vi "18-FindLeftRightExplode.vi"(10 "Explode Position":i32, 11 "Snailfish Number in in":string) -> (0 "Right Explosion":u64, 1 "Right Snailfish Number out":string, 2 "Left Explosion":u64, 3 "Left Snailfish Number out":string)   [LabVIEW 2019, in "18.lvlib"]
uses:
  18.lvlib
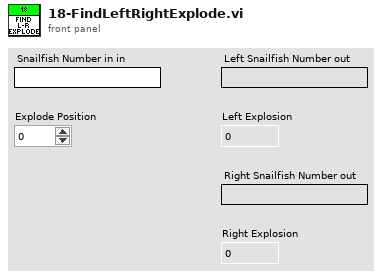
[diagram p1: front panel]
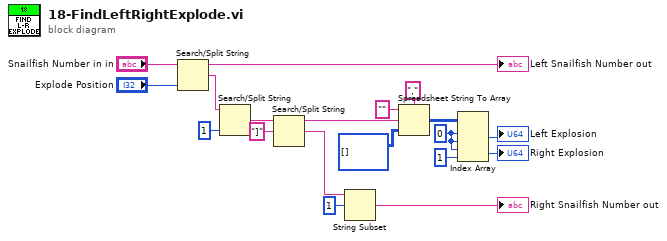
[diagram p0: block diagram]
diagram:
  w11 = 0 ("index (row)")
  n1 = Search/Split String(string="Snailfish Number in in", offset (0)="Explode Position") -> (substring before match=→"Left Snailfish Number out":string, match + rest of string=w14:string)  [unwired: 1 in, 1 out]
  n2 = Search/Split String(string=w14, offset (0)=1) -> (match + rest of string=w15:string)  [unwired: 1 in, 2 out]
  n3 = Search/Split String(string=w15, search string/char (-)="]") -> (substring before match=w6:string, match + rest of string=w3:string)  [unwired: 1 in, 1 out]
  n4 = String Subset(string=w3, offset (0)=1) -> (substring=→"Right Snailfish Number out":string)  [unwired: 1 in]
  n5 = Spreadsheet String To Array(delimiter (Tab)=",", format string="", spreadsheet string=w6, array type (2D Dbl)=u64[][] [] ("Position of Last Number")) -> (array=w10:u64[][])
  n6 = Index Array(array=w10, index (row) #1=w11, index (col) #1=w11, index (row) #2=w11, index (col) #2=1 ("disabled index (col)")) -> (element #1=→"Left Explosion":u64, element #2=→"Right Explosion":u64)
